vi "estimate covariance.vi"(9 "Q_k":T1=[[1.0, 0.0, 0.0], [0.0, 1.0, 0.0], [0.0, 0.0, 1.0]], 10 "Pk-1|k-1":T1, 11 "F_k":T1) -> (3 "Pk|k-1":T1)   [LabVIEW 2018]
uses:
  <vilib>/Analysis/Matrix/Datatypes/RealMatrix.ctl
  <vilib>/Analysis/baseanly.llb/Real A x B.vi
  <vilib>/Analysis/Matrix/Numeric/Add/Add - RM,RM.vi
  <vilib>/Analysis/Matrix/NI_Matrix.lvlib
  <vilib>/Analysis/NI_AALBase.lvlib
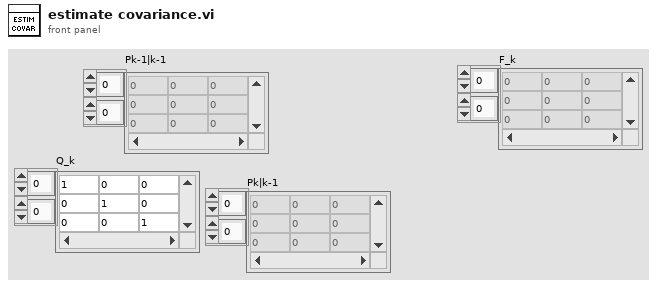
[diagram p1: front panel]
types:
  T1 = typedef "NI_Matrix.lvlib/RealMatrix.ctl" = dbl[][]
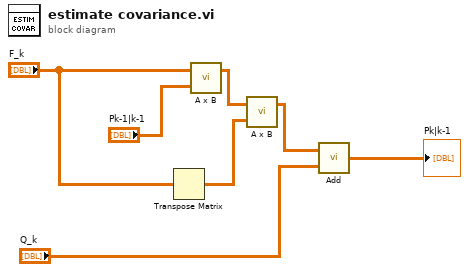
[diagram p0: block diagram]
diagram:
  n1 = Transpose Matrix(1:"F_k") -> (0:w4:T1)
  n2 = call-poly <vilib>:"A x B.vi"("B"="Pk-1|k-1", "A"="F_k") -> ("A x B"=w5:T1)  [unwired: 1 out]
  n3 = call-poly <vilib>:"A x B.vi"("B"=w4, "A"=w5) -> ("A x B"=w3:T1)  [unwired: 1 out]
  n4 = call-poly <vilib>:"Add.vi"("Real Matrix B"="Q_k", "Real Matrix A"=w3) -> ("A + B"=→"Pk|k-1":T1)
